vi "Preparation_strings_msgs.vi"(9 "Enum":T1, 10 "reference":refnum<vi>, 11 "Cluster in":refnum<vi>) -> (3 "Status":string="Take our chance")   [LabVIEW 2019]
uses:
  Enum_states.ctl
panel:
  out "error out":errorcluster
  in  "error in (no error)":errorcluster
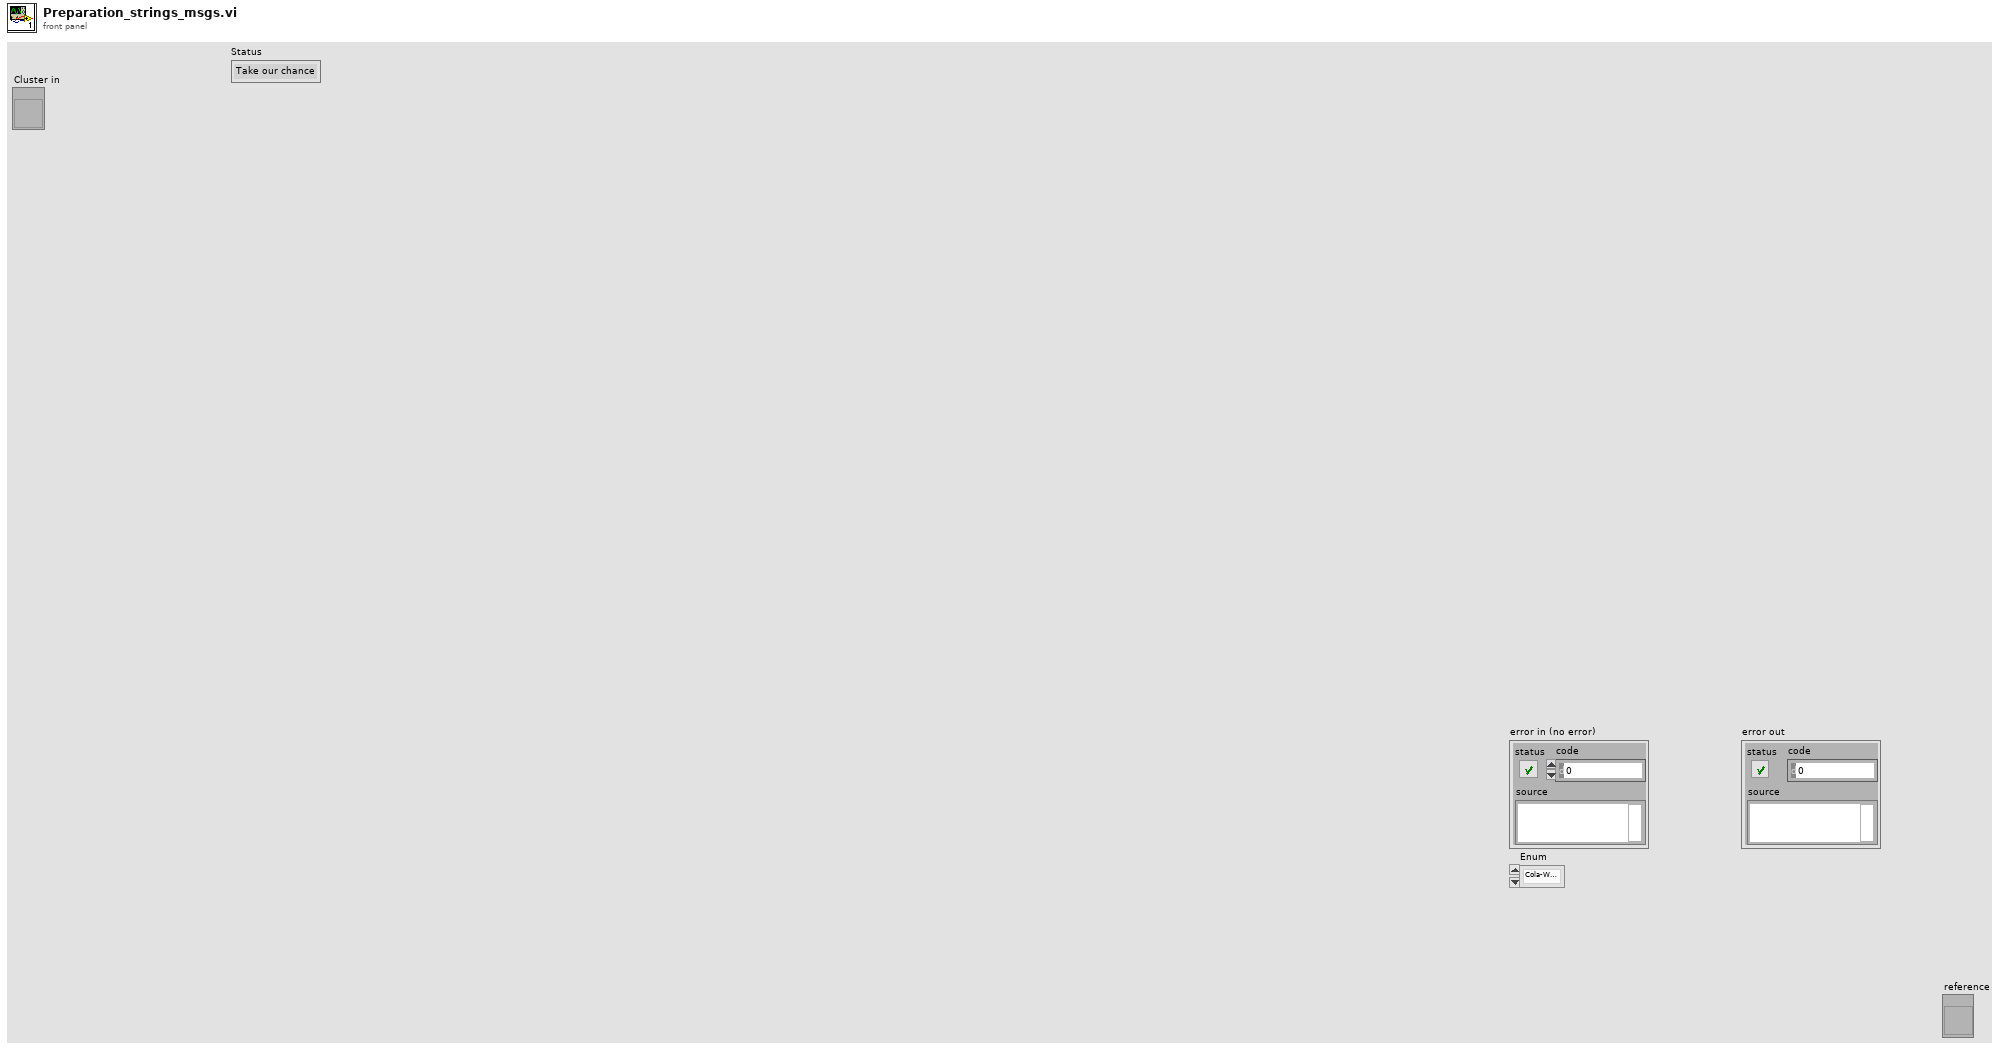
[diagram p1: front panel]
types:
  T1 = typedef "Enum_states.ctl" = enum16{"Cola-WaitMessage", "caipirinha", "whisky-sour", "whisky-cola", "water-juice", "water", "cola", "add0.5", "add1", "add2", "add5", "initialize", "OFF", "Admin mode", "Refill", "stop"}
  T2 = typedef "Control_typedef.ctl" = cluster{"Status":string, "Credit":string}
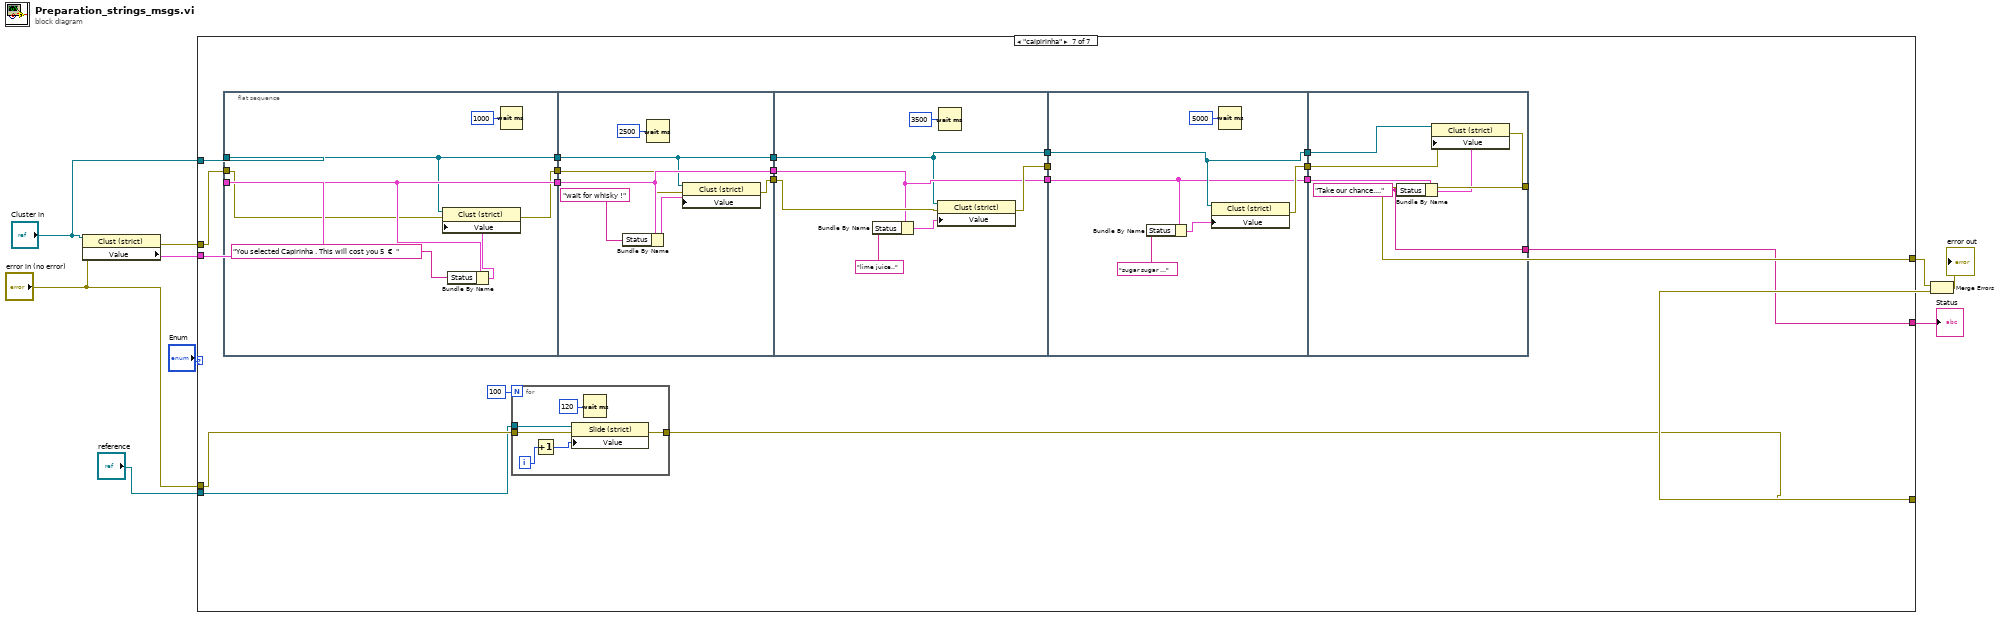
[diagram p0: block diagram]
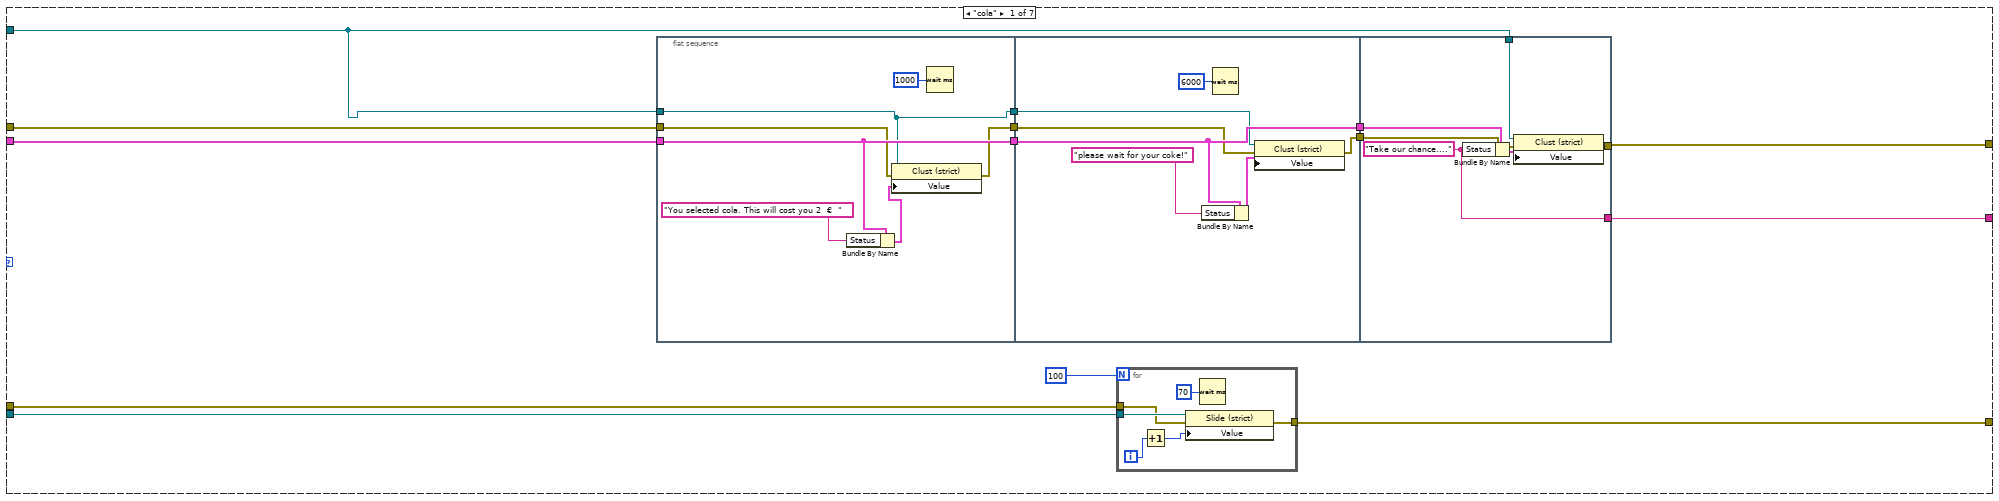
[diagram p2: hidden frame]
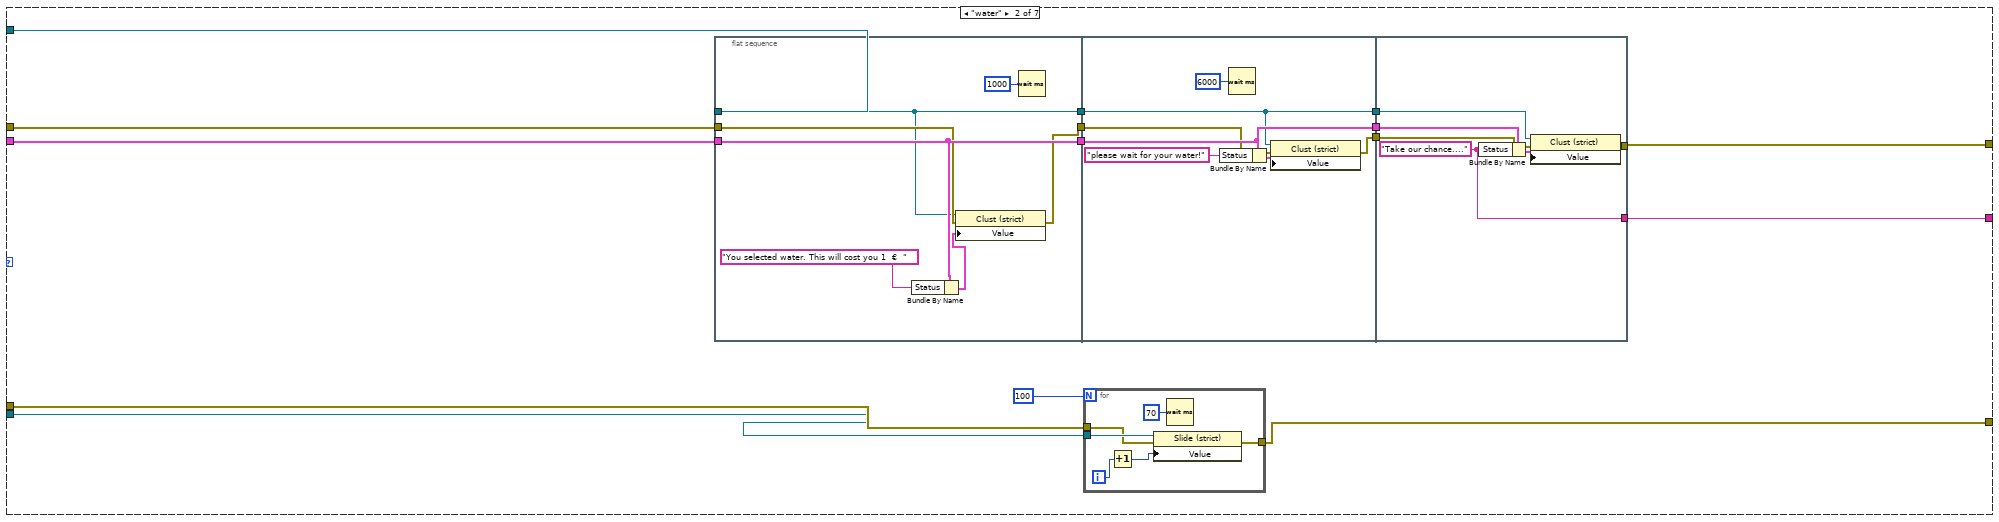
[diagram p3: hidden frame]
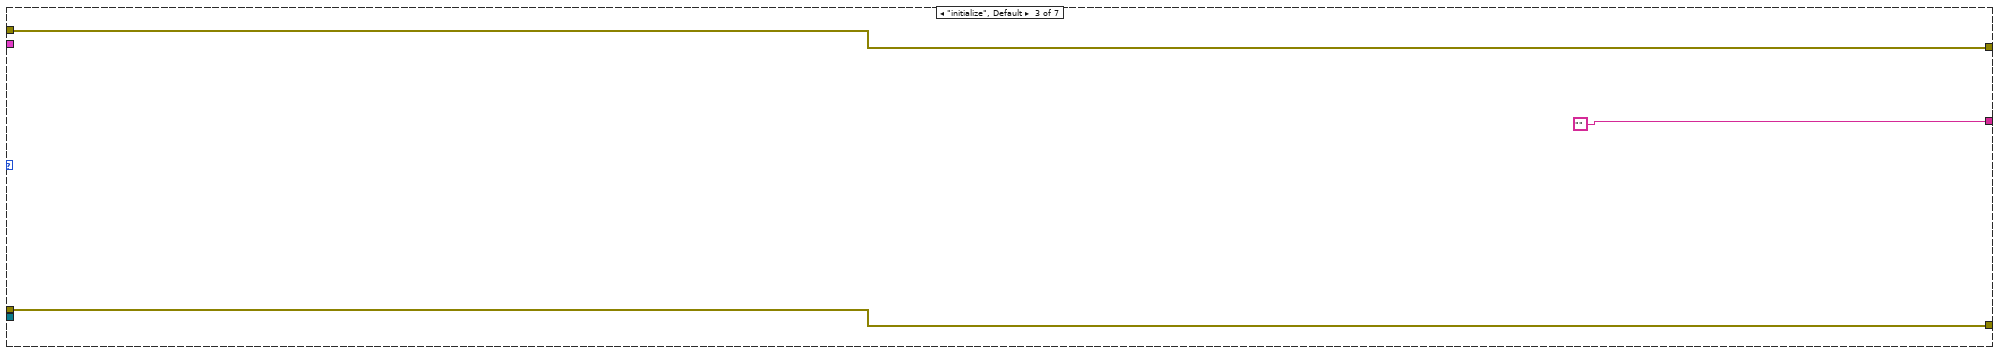
[diagram p4: hidden frame]
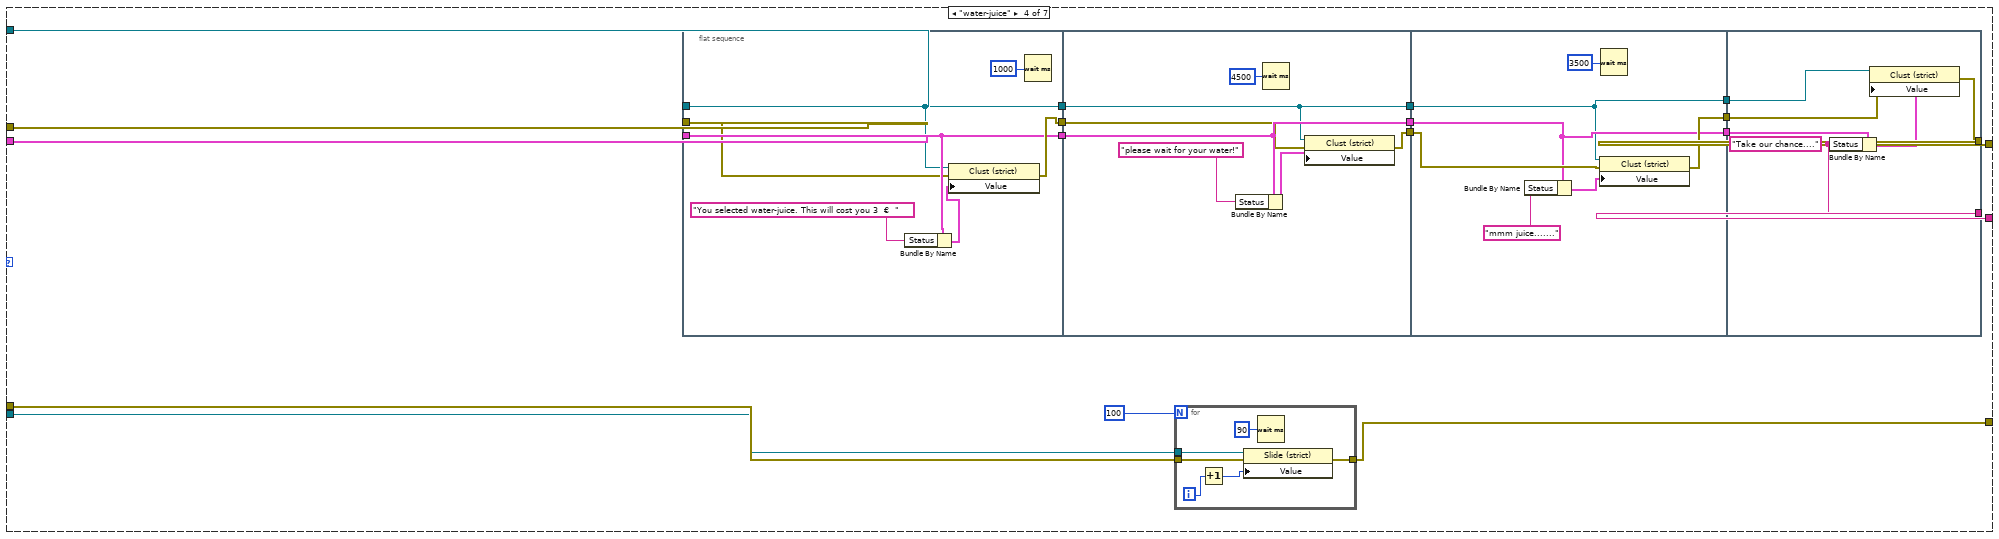
[diagram p5: hidden frame]
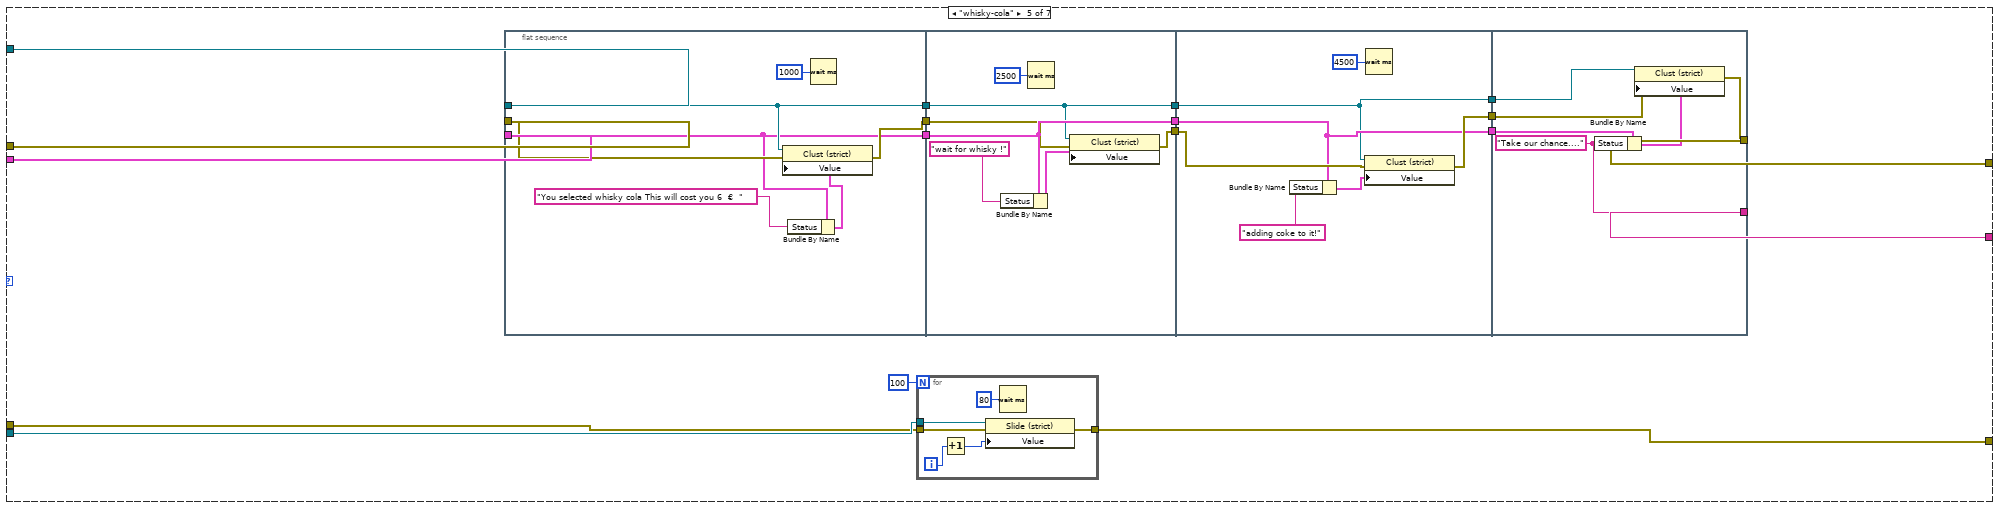
[diagram p6: hidden frame]
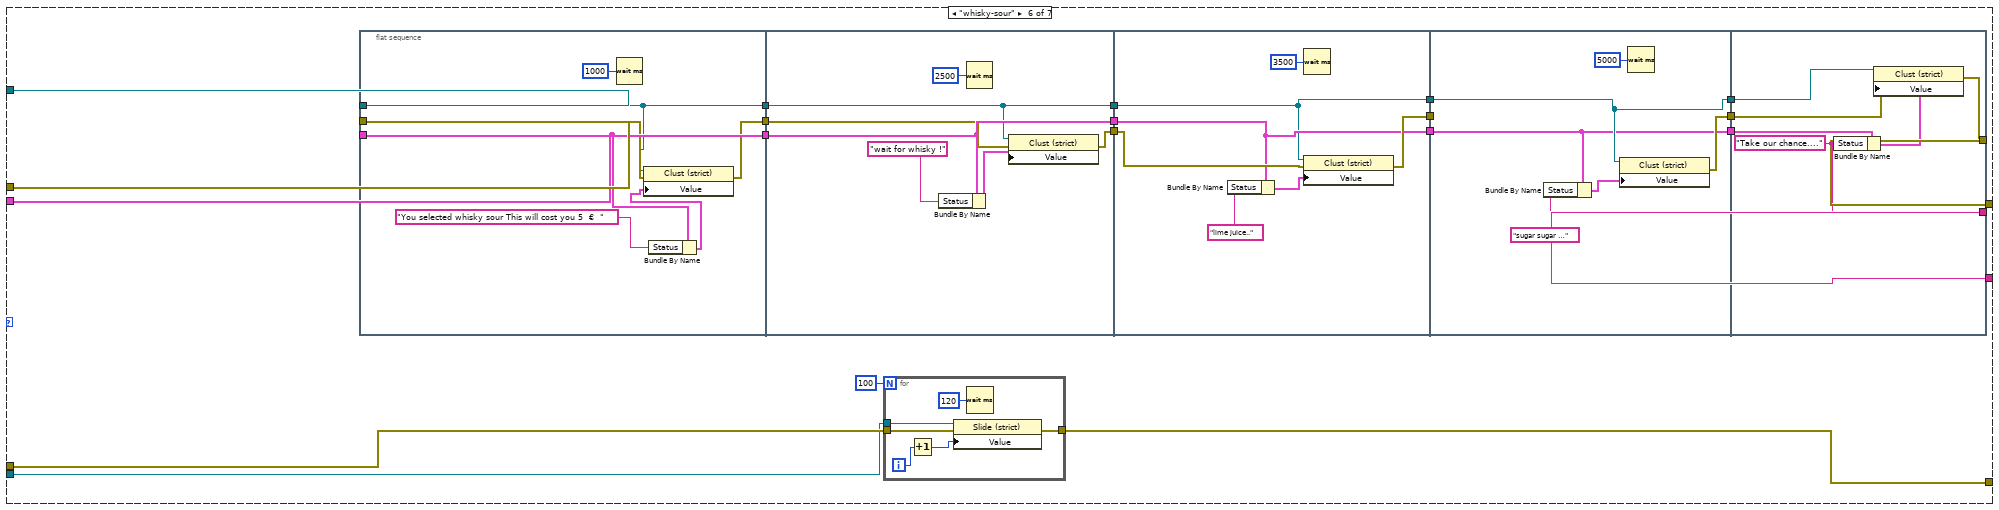
[diagram p7: hidden frame]
diagram:
  n1 = property class="Clust (strict)"(reference="Cluster in", error in="error in (no error)") -> (error out=w5:errorcluster, "Value"=w10:T2)  [unwired: 1 out]
  n2 = case shown="\"caipirinha\"" "Enum" {
    tunnel: w10 -> [w22 w62 _ w110 w155 w212 w267]
    tunnel: "Cluster in" -> [w21 w61 _ w112 w157 w214 w268]
    tunnel: [w20 w58 "" w108 w153 w210 w264] -> w8
    tunnel: "reference" -> [w19 w55 _ w98 w152 w202 w262]
    tunnel: "error in (no error)" -> [w17 w56 w92 w99 w151 w203 w263]
    tunnel: w5 -> [w16 w63 w94 w111 w156 w213 w266]
    tunnel: [w15 w59 w94 w109 w154 w211 w265] -> w4
    tunnel: [w14 w54 w92 w100 w150 w201 w261] -> w3
    frame "cola" {
      n3 = flat-sequence {
        tunnel: w16 -> [w34]
        tunnel: w21 -> [w32]
        tunnel: w22 -> [w35]
        tunnel: [w35] -> w13
        tunnel: [w33] -> w12
        tunnel: [w32] -> w11
        tunnel: [w41] -> w24
        tunnel: [w38] -> w23
        tunnel: w13 -> [w41]
        tunnel: w12 -> [w39]
        tunnel: w11 -> [w40]
        tunnel: w24 -> [w49]
        tunnel: w21 -> [w48]
        tunnel: [w47] -> w20
        tunnel: w23 -> [w46]
        tunnel: [w45] -> w15
        frame #0 {
          n4 = Bundle By Name(cluster=w35, "Status"="You selected cola. This will cost you 2  €  ") -> (w36:T2)
          n5 = property class="Clust (strict)"(reference=w32, error in=w34, "Value"=w36) -> (error out=w33:errorcluster)  [unwired: 1 out]
          n6 = Wait (ms)(milliseconds to wait=u32 1000) -> ()  [unwired: 1 out]
        }
        frame #1 {
          n7 = Bundle By Name(cluster=w41, "Status"="please wait for your coke!") -> (w43:T2)
          n8 = Wait (ms)(milliseconds to wait=u32 6000) -> ()  [unwired: 1 out]
          n9 = property class="Clust (strict)"(reference=w40, error in=w39, "Value"=w43) -> (error out=w38:errorcluster)  [unwired: 1 out]
        }
        frame #2 {
          w47 = "Take our chance...." ("Status")
          n10 = Bundle By Name(cluster=w49, "Status"=w47) -> (w50:T2)
          n11 = property class="Clust (strict)"(reference=w48, error in=w46, "Value"=w50) -> (error out=w45:errorcluster)  [unwired: 1 out]
        }
      }
      n12 = for {
        N: 100 -> [_]
        tunnel: w19 -> [w28]
        tunnel: w17 -> [w26]
        tunnel: [w25] -> w14
        i -> [w30]
        n13 = Increment(x=w30) -> (x+1=w27:i32)
        n14 = property on="Property Node" class="Slide (strict)"(reference=w28, error in=w26, "Value"=w27) -> (error out=w25:errorcluster)  [unwired: 1 out]
        n15 = Wait (ms)(milliseconds to wait=u32 70) -> ()  [unwired: 1 out]
      }
    }
    frame "water" {
      n16 = flat-sequence {
        tunnel: w63 -> [w75]
        tunnel: w61 -> [w74]
        tunnel: w62 -> [w76]
        tunnel: [w76] -> w53
        tunnel: [w74] -> w52
        tunnel: [w73] -> w51
        tunnel: [w82] -> w65
        tunnel: [w80] -> w64
        tunnel: [w79] -> w60
        tunnel: w53 -> [w82]
        tunnel: w52 -> [w79]
        tunnel: w51 -> [w81]
        tunnel: w65 -> [w90]
        tunnel: [w89] -> w58
        tunnel: w64 -> [w88]
        tunnel: [w87] -> w59
        tunnel: w60 -> [w86]
        frame #0 {
          n17 = Bundle By Name(cluster=w76, "Status"="You selected water. This will cost you 1  €  ") -> (w77:T2)
          n18 = property class="Clust (strict)"(reference=w74, error in=w75, "Value"=w77) -> (error out=w73:errorcluster)  [unwired: 1 out]
          n19 = Wait (ms)(milliseconds to wait=u32 1000) -> ()  [unwired: 1 out]
        }
        frame #1 {
          n20 = Bundle By Name(cluster=w82, "Status"="please wait for your water!") -> (w84:T2)
          n21 = Wait (ms)(milliseconds to wait=u32 6000) -> ()  [unwired: 1 out]
          n22 = property class="Clust (strict)"(reference=w79, error in=w81, "Value"=w84) -> (error out=w80:errorcluster)  [unwired: 1 out]
        }
        frame #2 {
          w89 = "Take our chance...." ("Status")
          n23 = Bundle By Name(cluster=w90, "Status"=w89) -> (w91:T2)
          n24 = property class="Clust (strict)"(reference=w86, error in=w88, "Value"=w91) -> (error out=w87:errorcluster)  [unwired: 1 out]
        }
      }
      n25 = for {
        N: 100 -> [_]
        tunnel: w55 -> [w69]
        tunnel: w56 -> [w67]
        tunnel: [w66] -> w54
        i -> [w71]
        n26 = Increment(x=w71) -> (x+1=w68:i32)
        n27 = property on="Property Node" class="Slide (strict)"(reference=w69, error in=w67, "Value"=w68) -> (error out=w66:errorcluster)  [unwired: 1 out]
        n28 = Wait (ms)(milliseconds to wait=u32 70) -> ()  [unwired: 1 out]
      }
    }
    frame "initialize", Default {
    }
    frame "water-juice" {
      n29 = flat-sequence {
        tunnel: w111 -> [w120]
        tunnel: w112 -> [w121]
        tunnel: w110 -> [w122]
        tunnel: [w121] -> w97
        tunnel: [w123] -> w96
        tunnel: [w122] -> w95
        tunnel: [w129] -> w107
        tunnel: [w127] -> w106
        tunnel: [w126] -> w105
        tunnel: w97 -> [w126]
        tunnel: w96 -> [w128]
        tunnel: w95 -> [w129]
        tunnel: w107 -> [w136]
        tunnel: w106 -> [w138]
        tunnel: w105 -> [w135]
        tunnel: [w137] -> w104
        tunnel: [w136] -> w103
        tunnel: [w135] -> w102
        tunnel: [w145] -> w108
        tunnel: [w144] -> w109
        tunnel: w104 -> [w143]
        tunnel: w103 -> [w142]
        tunnel: w102 -> [w141]
        frame #0 {
          n30 = Bundle By Name(cluster=w122, "Status"="You selected water-juice. This will cost you 3  €  ") -> (w124:T2)
          n31 = property class="Clust (strict)"(reference=w121, error in=w120, "Value"=w124) -> (error out=w123:errorcluster)  [unwired: 1 out]
          n32 = Wait (ms)(milliseconds to wait=u32 1000) -> ()  [unwired: 1 out]
        }
        frame #1 {
          n33 = Bundle By Name(cluster=w129, "Status"="please wait for your water!") -> (w131:T2)
          n34 = Wait (ms)(milliseconds to wait=u32 4500) -> ()  [unwired: 1 out]
          n35 = property class="Clust (strict)"(reference=w126, error in=w128, "Value"=w131) -> (error out=w127:errorcluster)  [unwired: 1 out]
        }
        frame #2 {
          n36 = Bundle By Name(cluster=w136, "Status"="mmm juice.......") -> (w133:T2)
          n37 = property class="Clust (strict)"(reference=w135, error in=w138, "Value"=w133) -> (error out=w137:errorcluster)  [unwired: 1 out]
          n38 = Wait (ms)(milliseconds to wait=u32 3500) -> ()  [unwired: 1 out]
        }
        frame #3 {
          w145 = "Take our chance...." ("Status")
          n39 = Bundle By Name(cluster=w142, "Status"=w145) -> (w140:T2)
          n40 = property class="Clust (strict)"(reference=w141, error in=w143, "Value"=w140) -> (error out=w144:errorcluster)  [unwired: 1 out]
        }
      }
      n41 = for {
        N: 100 -> [_]
        tunnel: [w115] -> w100
        tunnel: w99 -> [w114]
        tunnel: w98 -> [w113]
        i -> [w118]
        n42 = Increment(x=w118) -> (x+1=w116:i32)
        n43 = property on="Property Node" class="Slide (strict)"(reference=w113, error in=w114, "Value"=w116) -> (error out=w115:errorcluster)  [unwired: 1 out]
        n44 = Wait (ms)(milliseconds to wait=u32 90) -> ()  [unwired: 1 out]
      }
    }
    frame "whisky-cola" {
      n45 = flat-sequence {
        tunnel: w156 -> [w174]
        tunnel: w157 -> [w172]
        tunnel: w155 -> [w171]
        tunnel: [w171] -> w148
        tunnel: [w172] -> w147
        tunnel: [w173] -> w146
        tunnel: [w180] -> w163
        tunnel: [w178] -> w162
        tunnel: [w177] -> w161
        tunnel: w148 -> [w180]
        tunnel: w147 -> [w177]
        tunnel: w146 -> [w179]
        tunnel: w163 -> [w187]
        tunnel: w162 -> [w189]
        tunnel: w161 -> [w186]
        tunnel: [w188] -> w160
        tunnel: [w187] -> w159
        tunnel: [w186] -> w158
        tunnel: [w196] -> w153
        tunnel: [w195] -> w154
        tunnel: w160 -> [w194]
        tunnel: w159 -> [w193]
        tunnel: w158 -> [w192]
        frame #0 {
          n46 = Bundle By Name(cluster=w171, "Status"="You selected whisky cola This will cost you 6  €  ") -> (w175:T2)
          n47 = property class="Clust (strict)"(reference=w172, error in=w174, "Value"=w175) -> (error out=w173:errorcluster)  [unwired: 1 out]
          n48 = Wait (ms)(milliseconds to wait=u32 1000) -> ()  [unwired: 1 out]
        }
        frame #1 {
          n49 = Bundle By Name(cluster=w180, "Status"="wait for whisky !") -> (w182:T2)
          n50 = Wait (ms)(milliseconds to wait=u32 2500) -> ()  [unwired: 1 out]
          n51 = property class="Clust (strict)"(reference=w177, error in=w179, "Value"=w182) -> (error out=w178:errorcluster)  [unwired: 1 out]
        }
        frame #2 {
          n52 = Bundle By Name(cluster=w187, "Status"="adding coke to it!") -> (w184:T2)
          n53 = property class="Clust (strict)"(reference=w186, error in=w189, "Value"=w184) -> (error out=w188:errorcluster)  [unwired: 1 out]
          n54 = Wait (ms)(milliseconds to wait=u32 4500) -> ()  [unwired: 1 out]
        }
        frame #3 {
          w196 = "Take our chance...." ("Status")
          n55 = Bundle By Name(cluster=w193, "Status"=w196) -> (w191:T2)
          n56 = property class="Clust (strict)"(reference=w192, error in=w194, "Value"=w191) -> (error out=w195:errorcluster)  [unwired: 1 out]
        }
      }
      n57 = for {
        N: 100 -> [_]
        tunnel: [w166] -> w150
        tunnel: w151 -> [w165]
        tunnel: w152 -> [w164]
        i -> [w169]
        n58 = Increment(x=w169) -> (x+1=w167:i32)
        n59 = property on="Property Node" class="Slide (strict)"(reference=w164, error in=w165, "Value"=w167) -> (error out=w166:errorcluster)  [unwired: 1 out]
        n60 = Wait (ms)(milliseconds to wait=u32 80) -> ()  [unwired: 1 out]
      }
    }
    frame "whisky-sour" {
      n61 = flat-sequence {
        tunnel: w213 -> [w227]
        tunnel: w214 -> [w225]
        tunnel: w212 -> [w228]
        tunnel: [w228] -> w199
        tunnel: [w225] -> w198
        tunnel: [w226] -> w197
        tunnel: [w234] -> w217
        tunnel: [w232] -> w216
        tunnel: [w231] -> w215
        tunnel: w199 -> [w234]
        tunnel: w198 -> [w231]
        tunnel: w197 -> [w233]
        tunnel: w217 -> [w241]
        tunnel: w216 -> [w243]
        tunnel: w215 -> [w240]
        tunnel: [w242] -> w209
        tunnel: [w241] -> w207
        tunnel: [w240] -> w206
        tunnel: w209 -> [_]
        tunnel: [w248] -> w208
        tunnel: w207 -> [w246]
        tunnel: w206 -> [w247]
        tunnel: [w247] -> w205
        tunnel: [w246] -> w204
        tunnel: [w256] -> w210
        tunnel: [w255] -> w211
        tunnel: w208 -> [w254]
        tunnel: w205 -> [w252]
        tunnel: w204 -> [w253]
        frame #0 {
          n62 = Wait (ms)(milliseconds to wait=u32 1000) -> ()  [unwired: 1 out]
          n63 = Bundle By Name(cluster=w228, "Status"="You selected whisky sour This will cost you 5  €  ") -> (w229:T2)
          n64 = property class="Clust (strict)"(reference=w225, error in=w227, "Value"=w229) -> (error out=w226:errorcluster)  [unwired: 1 out]
        }
        frame #1 {
          n65 = Bundle By Name(cluster=w234, "Status"="wait for whisky !") -> (w236:T2)
          n66 = Wait (ms)(milliseconds to wait=u32 2500) -> ()  [unwired: 1 out]
          n67 = property class="Clust (strict)"(reference=w231, error in=w233, "Value"=w236) -> (error out=w232:errorcluster)  [unwired: 1 out]
        }
        frame #2 {
          n68 = Bundle By Name(cluster=w241, "Status"="lime juice..") -> (w238:T2)
          n69 = property class="Clust (strict)"(reference=w240, error in=w243, "Value"=w238) -> (error out=w242:errorcluster)  [unwired: 1 out]
          n70 = Wait (ms)(milliseconds to wait=u32 3500) -> ()  [unwired: 1 out]
        }
        frame #3 {
          n71 = Bundle By Name(cluster=w246, "Status"="sugar sugar …") -> (w249:T2)
          n72 = property class="Clust (strict)"(reference=w247, "Value"=w249) -> (error out=w248:errorcluster)  [unwired: 1 in, 1 out]
          n73 = Wait (ms)(milliseconds to wait=u32 5000) -> ()  [unwired: 1 out]
        }
        frame #4 {
          w256 = "Take our chance...." ("Status")
          n74 = Bundle By Name(cluster=w253, "Status"=w256) -> (w251:T2)
          n75 = property class="Clust (strict)"(reference=w252, error in=w254, "Value"=w251) -> (error out=w255:errorcluster)  [unwired: 1 out]
        }
      }
      n76 = for {
        N: 100 -> [_]
        tunnel: [w220] -> w201
        tunnel: w203 -> [w219]
        tunnel: w202 -> [w218]
        i -> [w223]
        n77 = Increment(x=w223) -> (x+1=w221:i32)
        n78 = property on="Property Node" class="Slide (strict)"(reference=w218, error in=w219, "Value"=w221) -> (error out=w220:errorcluster)  [unwired: 1 out]
        n79 = Wait (ms)(milliseconds to wait=u32 120) -> ()  [unwired: 1 out]
      }
    }
    frame "caipirinha" {
      n80 = flat-sequence {
        tunnel: w266 -> [w285]
        tunnel: w268 -> [w287]
        tunnel: w267 -> [w288]
        tunnel: [w288] -> w259
        tunnel: [w287] -> w258
        tunnel: [w286] -> w257
        tunnel: [w294] -> w277
        tunnel: [w292] -> w276
        tunnel: [w291] -> w275
        tunnel: w259 -> [w294]
        tunnel: w258 -> [w291]
        tunnel: w257 -> [w293]
        tunnel: w277 -> [w301]
        tunnel: w276 -> [w303]
        tunnel: w275 -> [w300]
        tunnel: [w302] -> w274
        tunnel: [w301] -> w273
        tunnel: [w300] -> w272
        tunnel: w274 -> [_]
        tunnel: [w308] -> w271
        tunnel: w273 -> [w306]
        tunnel: w272 -> [w307]
        tunnel: [w307] -> w270
        tunnel: [w306] -> w269
        tunnel: [w316] -> w264
        tunnel: [w315] -> w265
        tunnel: w271 -> [w314]
        tunnel: w270 -> [w312]
        tunnel: w269 -> [w313]
        frame #0 {
          n81 = Bundle By Name(cluster=w288, "Status"="You selected Capirinha . This will cost you 5  €  ") -> (w289:T2)
          n82 = property class="Clust (strict)"(reference=w287, error in=w285, "Value"=w289) -> (error out=w286:errorcluster)  [unwired: 1 out]
          n83 = Wait (ms)(milliseconds to wait=u32 1000) -> ()  [unwired: 1 out]
        }
        frame #1 {
          n84 = Bundle By Name(cluster=w294, "Status"="wait for whisky !") -> (w296:T2)
          n85 = Wait (ms)(milliseconds to wait=u32 2500) -> ()  [unwired: 1 out]
          n86 = property class="Clust (strict)"(reference=w291, error in=w293, "Value"=w296) -> (error out=w292:errorcluster)  [unwired: 1 out]
        }
        frame #2 {
          n87 = Bundle By Name(cluster=w301, "Status"="lime juice..") -> (w298:T2)
          n88 = property class="Clust (strict)"(reference=w300, error in=w303, "Value"=w298) -> (error out=w302:errorcluster)  [unwired: 1 out]
          n89 = Wait (ms)(milliseconds to wait=u32 3500) -> ()  [unwired: 1 out]
        }
        frame #3 {
          n90 = Bundle By Name(cluster=w306, "Status"="sugar sugar …") -> (w309:T2)
          n91 = property class="Clust (strict)"(reference=w307, "Value"=w309) -> (error out=w308:errorcluster)  [unwired: 1 in, 1 out]
          n92 = Wait (ms)(milliseconds to wait=u32 5000) -> ()  [unwired: 1 out]
        }
        frame #4 {
          w316 = "Take our chance...." ("Status")
          n93 = Bundle By Name(cluster=w313, "Status"=w316) -> (w311:T2)
          n94 = property class="Clust (strict)"(reference=w312, error in=w314, "Value"=w311) -> (error out=w315:errorcluster)  [unwired: 1 out]
        }
      }
      n95 = for {
        N: 100 -> [_]
        tunnel: [w280] -> w261
        tunnel: w263 -> [w279]
        tunnel: w262 -> [w278]
        i -> [w283]
        n96 = Increment(x=w283) -> (x+1=w281:i32)
        n97 = property on="Property Node" class="Slide (strict)"(reference=w278, error in=w279, "Value"=w281) -> (error out=w280:errorcluster)  [unwired: 1 out]
        n98 = Wait (ms)(milliseconds to wait=u32 120) -> ()  [unwired: 1 out]
      }
    }
  }
  "Status" <- w8
  n99 = Merge Errors(w4, w3) -> (→"error out":errorcluster)
